vi "NI5112.constructor.vi"(0 "name":string, 2 "data in":string, 5 "error in(no error)":errorcluster) -> (14 "i ref out":refnum<vi>, 16 "data out":string, 19 "error out":errorcluster)   [LabVIEW 2014, in "NI5112.lvlib"]
doc: "This is the constructor of a class.\n\nLicense Agreement for this software:\n\nCopyright (C)\nGesellschaft für Schwerionenforschung, GSI\nPlanckstr. 1\n64291 Darmstadt\nGermany\n\nContact: D.Beck@gsi.de \n\nThis program is free software; you can redistribute it and/or modify it under the terms of the \nGNU General Public License as published by the Free Software Foundation; either version 2 of \nthe license, or (at your option) any later version.\n\nThis program is distributed in the hope that it will be useful, but WITHOUT ANY WARRANTY; \nwithout even the implied warranty of MERCHANTABILITY or FITNESS FOR A PARTICULAR PURPOSE. See the GNU General License for more details (http://www.gnu.org).\n\nGesellschaft für Schwerionenforschung, GSI\nPlanckstr. 1, 64291 Darmstadt, Germany\nFor all questions and ideas contact: M.Richter@gsi.de, H.Brand@gsi.de or D.Beck@gsi.de.\nLast update: 16-JUN-2004"
uses:
  NI5112.lvlib
  CSCore/BaseProcess/BaseProcess.lvlib
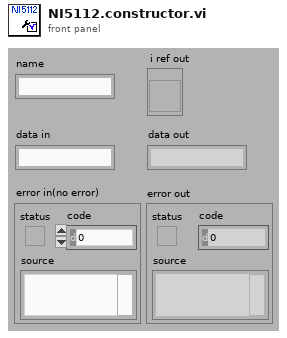
[diagram p1: front panel]
types:
  T1 = enum16{"SetAttribute", "GetAttribute", "CreateAttribute", "DestroyAttribute", "DestroyAllAtributes"}
  T2 = typedef "NI5112.lvlib/NI5112.i attribute.ctl" = cluster{"HWChannel":string, "instrument handle":refnum<k15>, "BinWidth":dbl, "vertical offset":dbl, "vertical range":dbl, "DataBPR":i32, "5112BPR":i32, "FullSpeed":bool, "discrLevel":dbl, "DoDiscr":bool, "VerCoupling":string}
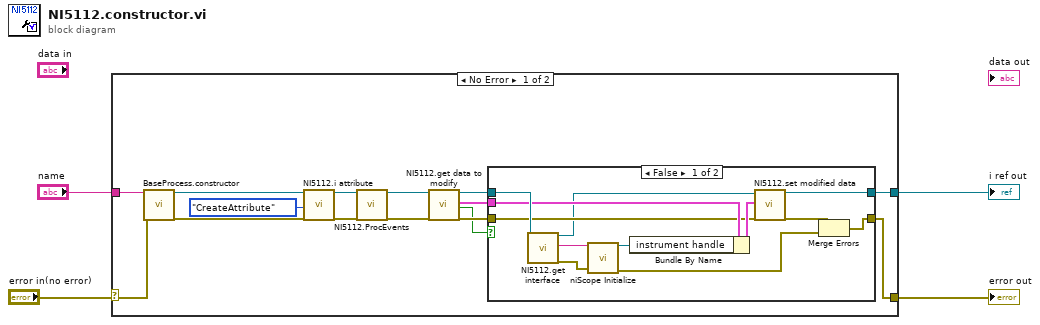
[diagram p0: block diagram]
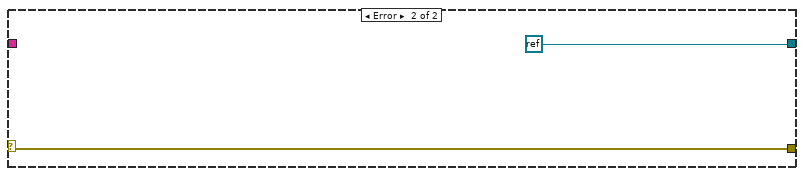
[diagram p3: hidden frame]
diagram:
  n1 = case shown="No Error" "error in(no error)" {
    selector: "error in(no error)" -> [w13 w35]
    tunnel: "name" -> [w16 _]
    tunnel: [w6 refnum<k0> refnum] -> w3
    tunnel: [w5 w35] -> w2
    frame No Error {
      n2 = call "BaseProcess.constructor.vi"("name"=w16, "error in (no error)"=w13) -> ("i ref out"=w19:refnum<vi>, "error out"=w18:errorcluster)  [unwired: 15 in, 1 out]
      n3 = call "NI5112.i attribute.vi"("VI Refnum"=w19, "Action"=T1."CreateAttribute", "error in (no error)"=w18) -> ("VI Refnum out"=w15:refnum<vi>, "error out"=w14:errorcluster)  [unwired: 14 in, 1 out]
      n4 = call "NI5112.ProcEvents.vi"("i ref in"=w15, "error in"=w14) -> ("i ref out"=w7:refnum<vi>, "error out"=w8:errorcluster)  [unwired: 16 in]
      n5 = call "NI5112.get data to modify.vi"("i ref in"=w7, "error in (no error)"=w8) -> ("i ref out"=w12:refnum<vi>, "i attribute"=w10:T2, "timed out"=w9:bool, "error out"=w11:errorcluster)  [unwired: 14 in]
      n6 = case shown="False" w9 {
        tunnel: [w24 w32] -> w5
        tunnel: [w31 w33] -> w6
        tunnel: w12 -> [w28 w33]
        tunnel: w11 -> [w25 w32]
        tunnel: w10 -> [w27 _]
        frame False {
          n7 = call "NI5112.get interface.vi"("i ref in"=w28) -> ("i ref out"=w21:refnum<vi>, "channel name"=w26:string, "error out"=w20:errorcluster)  [unwired: 15 in, 1 out]
          n8 = call <instrlib>:"niScope Initialize.vi"("resource name"=w26, "error in"=w20) -> ("instrument handle"=w29:refnum<k15>, "error out"=w22:errorcluster)  [unwired: 12 in]
          n9 = Bundle By Name(cluster=w27, "instrument handle"=w29) -> (w30:T2)
          n10 = call "NI5112.set modified data.vi"("i ref in"=w21, "i attribute"=w30, "error in (no error)"=w25) -> ("i ref out"=w31:refnum<vi>, "error out"=w23:errorcluster)  [unwired: 15 in]
          n11 = Merge Errors(w23, w22) -> (w24:errorcluster)
        }
        frame True {
        }
      }
    }
    frame Error {
    }
  }
  "i ref out" <- w3
  "error out" <- w2
